vi "merge_channels.vi"(7 "number of channels":i32, 8 "error in (no error)":errorcluster, 9 "FIFO_2":u32[](array[numeric]), 10 "FIFO_1":u32[](array[numeric]), 11 "FPGAWrapperRK120511Fiber_Spiral in":refnum<class "FPGAWrapperRK110512Fiber_Spiral.lvclass">) -> (0 "error out":errorcluster, 2 "channels raw data block":T1, 3 "FPGAWrapperRK120511Fiber_Spiral out":refnum<class "FPGAWrapperRK110512Fiber_Spiral.lvclass">)   [LabVIEW 2010, in "FPGAWrapperRK110512Fiber_Spiral.lvclass"]
uses:
  FPGAWrapperRK110512Fiber_Spiral.lvclass
  common/arrays/pixel_raw_data_array.ctl
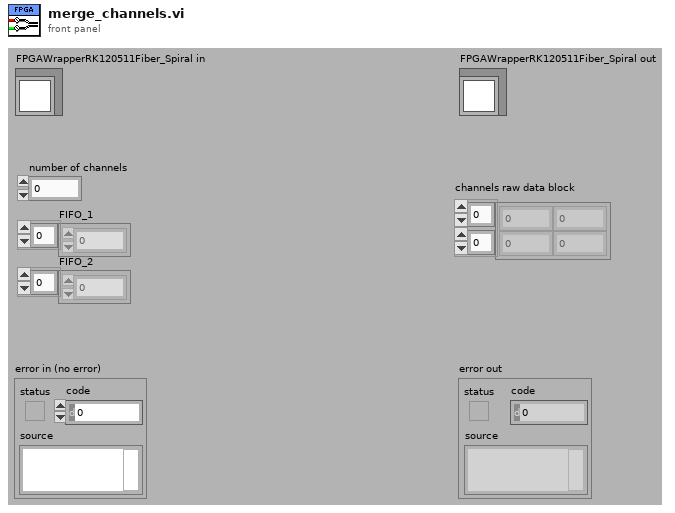
[diagram p1: front panel]
types:
  T1 = typedef "pixel_raw_data_array.ctl" = dbl[][]
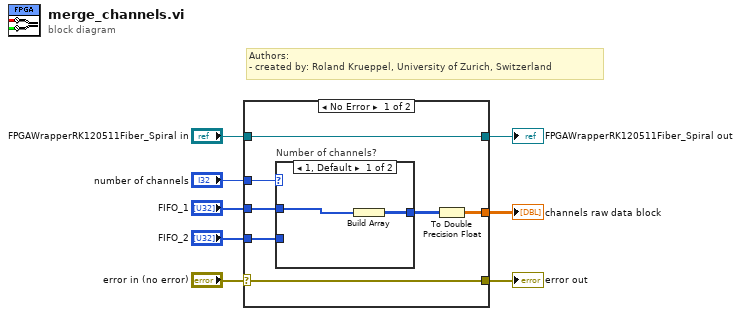
[diagram p0: block diagram]
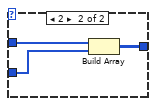
[diagram p2: hidden frame]
diagram:
  # "Authors: \n- created by: Roland Krueppel, University of Zurich, Switzerland"
  n1 = case shown="No Error" "error in (no error)" {
    selector: "error in (no error)" -> [w14 w22]
    tunnel: [w14 w22] -> w7
    tunnel: [w15 w21] -> w5
    tunnel: "FPGAWrapperRK120511Fiber_Spiral in" -> [w15 w21]
    tunnel: "number of channels" -> [w13 _]
    tunnel: "FIFO_1" -> [w12 _]
    tunnel: "FIFO_2" -> [w11 _]
    tunnel: [w9 _] -> w1
    frame No Error {
      n2 = case "Number of channels?" shown="1, Default" w13 {
        tunnel: w12 -> [w16 w19]
        tunnel: [w17 w20] -> w10
        tunnel: w11 -> [_ w18]
        frame 1, Default {
          n3 = Build Array(w16) -> (w17:u32[][])
        }
        frame 2 {
          n4 = Build Array(w19, w18) -> (w20:u32[][])
        }
      }
      n5 = To Double Precision Float(number=w10) -> (double precision float=w9:dbl[][])
    }
    frame Error {
    }
  }
  "error out" <- w7
  "FPGAWrapperRK120511Fiber_Spiral out" <- w5
  "channels raw data block" <- w1
